vi "HasMotionError.vi"(0 "System no.":i32, 2 "Axes to check":string[](array[string]), 5 "error in (no error)":errorcluster) -> (14 "Motion Error":bool, 19 "error out":errorcluster)   [LabVIEW 2026]
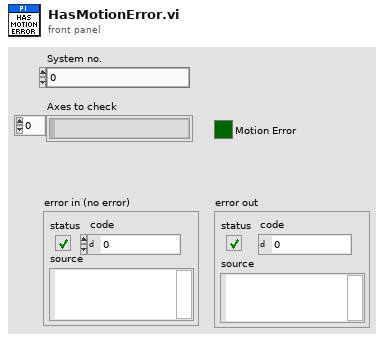
[diagram p1: front panel]
types:
  T1 = typedef "Syntax.ctl" = enum16{"GCS 1.0", "GCS 2.0", "GCS 3.0"}
  T2 = typedef "Status.ctl" = cluster{"Element":string, "Status bits":bool[]}
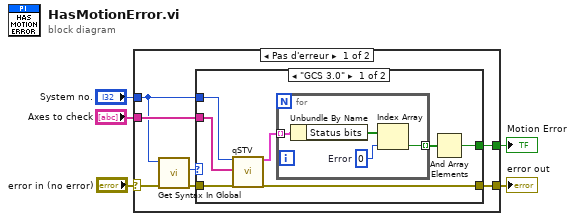
[diagram p0: block diagram]
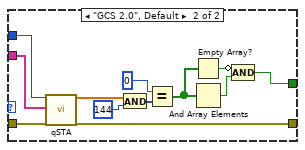
[diagram p2: hidden frame]
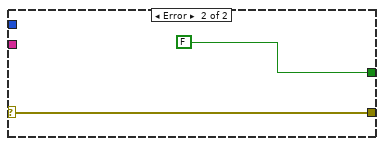
[diagram p3: hidden frame]
diagram:
  n1 = case shown="Pas d'erreur" "error in (no error)" {
    selector: "error in (no error)" -> [w6 w37]
    tunnel: [w12 w37] -> w5
    tunnel: "Axes to check" -> [w11 _]
    tunnel: "System no." -> [w8 _]
    tunnel: [w7 FALSE] -> w2
    frame No Error {
      n2 = call "Get Syntax In Global.vi"("error in"=w6, "System no."=w8) -> ("error out"=w10:errorcluster, "Syntax"=w9:T1)  [unwired: 8 in]
      n3 = case shown="\"GCS 3.0\"" w9 {
        tunnel: w8 -> [w19 w33]
        tunnel: w10 -> [w18 w28]
        tunnel: [w17 w35] -> w12
        tunnel: w11 -> [w15 w34]
        tunnel: [w13 w29] -> w7
        frame "GCS 3.0" {
          n4 = call "qSTV.vi"("System no."=w19, "Status Type"=w15, "error in"=w18) -> ("Status Array"=w16:T2[], "error out"=w17:errorcluster)  [unwired: 15 in]
          n5 = for {
            tunnel: w16 -> [w23] mode=indexing
            tunnel: [w20] -> w14 mode=indexing
            w21 = 0  # Error
            n6 = Unbundle By Name(w23) -> ("Status bits"=w22:bool[])
            n7 = Index Array(array=w22, index=w21) -> (element=w20:bool)
          }
          n8 = And Array Elements(Boolean array=w14) -> (logical AND=w13:bool)
        }
        frame "GCS 2.0", Default {
          n9 = call "qSTA.vi"("System no."=w33, "Axes to query"=w34, "error in"=w28) -> ("Axis status"=w26:dbl[], "error out"=w35:errorcluster)  [unwired: 2 in, 13 out]
          n10 = And(x=w26, y=u32 144) -> (x .and. y?=w24:i32[])
          n11 = Equal?(x=0 ("y"), y=w24) -> (x = y?=w30:bool[])
          n12 = Empty Array?(array=w30) -> (empty?=w31:bool)
          n13 = And Array Elements(Boolean array=w30) -> (logical AND=w32:bool)
          n14 = Compound Arithmetic op=AND(invert w31, w32) -> (w29:bool)
        }
      }
    }
    frame Error {
    }
  }
  "error out" <- w5
  "Motion Error" <- w2
